vi "DAQmx Timing (Burst Import Clock).vi"(0 "task/channels in":refnum<k21>, 1 "sample mode":i32(ring)=10178 items=["Finite Samples"=10178, "Continuous Samples"=10123, "Hardware Timed Single Point"=12522], 2 "samples per channel":i32=1000, 5 "sample clock rate":dbl=1000.0, 7 "sample clock source":tag, 9 "sample clock active edge":i32(ring)=10280 items=["Rising"=10280, "Falling"=10171], 11 "error in":errorcluster, 12 "pause when":i32(ring)=10192 items=["High"=10192, "Low"=10214], 13 "ready for transfer event active level":i32(ring)=10095 items=["Active High"=10095, "Active Low"=10096]) -> (4 "task out":refnum<k21>, 15 "error out":errorcluster)   [LabVIEW 2011]
doc: "Configures when the DAQ device transfers data to a peripheral device, using an imported sample clock to control burst handshake timing."
uses:
  C:/Program Files/National Instruments/LabVIEW 2011/resource/objmgr/daqmx.rc
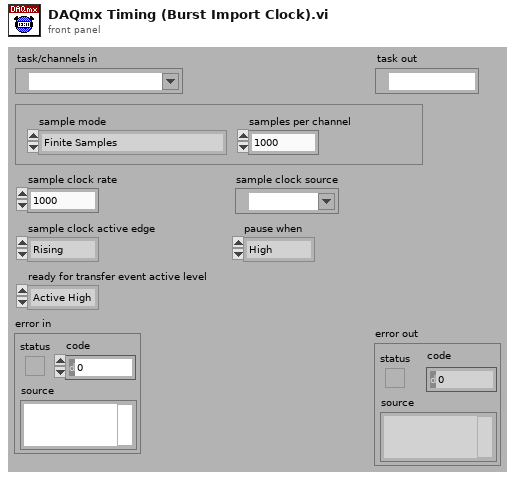
[diagram p1: front panel]
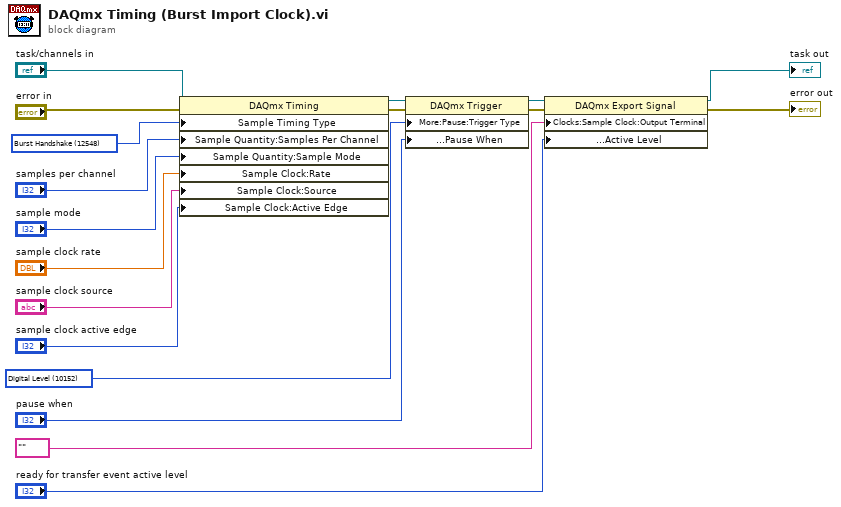
[diagram p0: block diagram]
diagram:
  w3 = 10152 items=["Analog Level"=10101, "Analog Window"=10103, "Digital Level"=10152, "None"=10230] ("Pause.TrigType")
  w14 = 12548 items=["Sample Clock"=10388, "Burst Handshake"=12548, "Handshake"=10389, "Implicit"=10451, "On Demand"=10390, "Change Detection"=12504] ("SampTimingType")
  n1 = property class="DAQmx Timing"(reference="task/channels in", error in="error in", "Sample Timing Type"=w14, "Sample Quantity:Samples Per Channel"="samples per channel", "Sample Quantity:Sample Mode"="sample mode", "Sample Clock:Rate"="sample clock rate", "Sample Clock:Source"="sample clock source", "Sample Clock:Active Edge"="sample clock active edge") -> (reference out=w10:refnum<k21>, error out=w9:errorcluster)
  n2 = property class="DAQmx Trigger"(reference=w10, error in=w9, "More:Pause:Trigger Type"=w3, "More:Pause:Digital Level:Pause When"="pause when") -> (reference out=w7:refnum<k21>, error out=w8:errorcluster)
  n3 = property class="DAQmx Export Signal"(reference=w7, error in=w8, "Clocks:Sample Clock:Output Terminal"=tag "" ("SampClk.OutputTerm"), "Events:Ready For Transfer Event:Level:Active Level"="ready for transfer event active level") -> (reference out=→"task out":refnum<k21>, error out=→"error out":errorcluster)
